vi "Pockels Cal-Calibration case logic.vi"(4 "Voltage %":u16[](array[numeric])=[0, 5, 10, 15, 20, 25, 30, 35, 40, 45, 50, 55, 60, 65, 70, 75, 80, 85, 90, 95, 100], 6 "Pockels calibration voltage steps sequence":dbl[](array[numeric])=[0.0, 0.05, 0.1, 0.15000000000000002, 0.2, 0.25, 0.3, 0.35, 0.39999999999999997, 0.44999999999999996, 0.49999999999999994, 0.5499999999999999, 0.6, 0.65, 0.7000000000000001, 0.7500000000000001, 0.8000000000000002, 0.8500000000000002, 0.9000000000000002, 0.9500000000000003, 1.0000000000000002], 7 "Number of objectives + 1":i32, 10 "Objective's name":string, 11 "Parent FOR loop's index":i32) -> (0 "error out":errorcluster, 2 "Timed out or errored out":bool, 3 "Cancel & Exit":bool, 5 "Output Strings":string[](array[string]))   [LabVIEW 2020]
panel:
  out "Cal indexes":i32[](array[numeric])
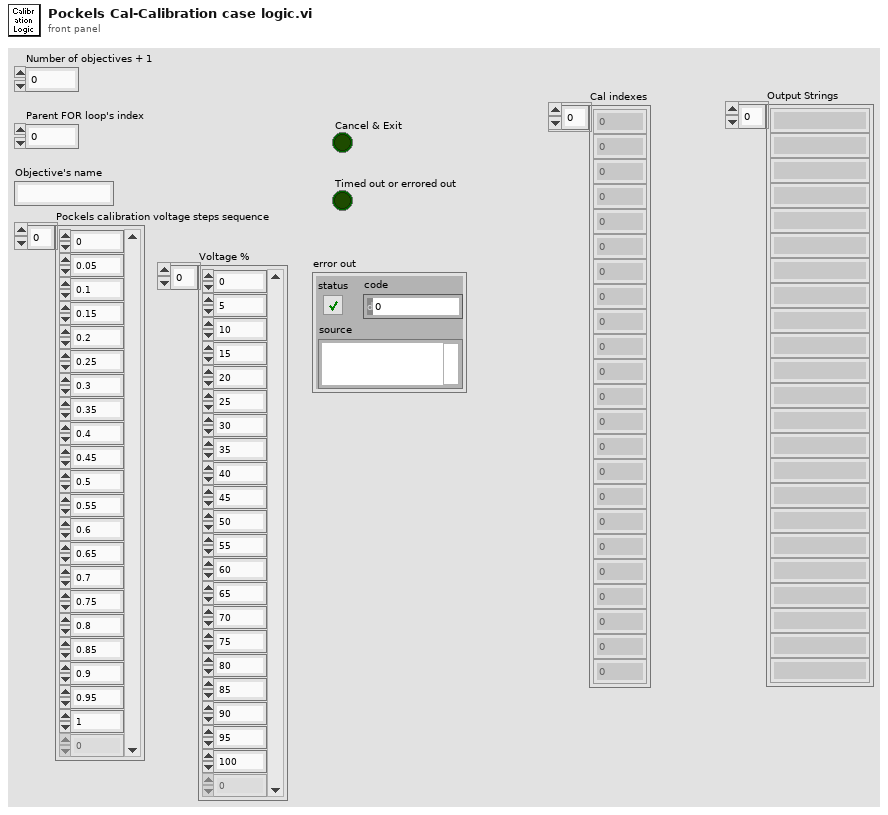
[diagram p1: front panel]
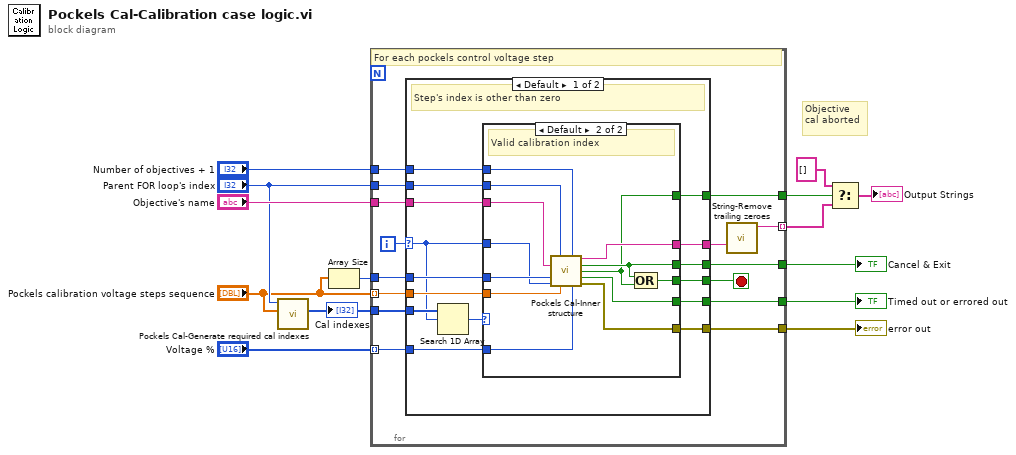
[diagram p0: block diagram]
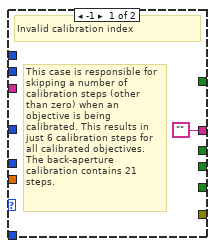
[diagram p2: hidden frame]
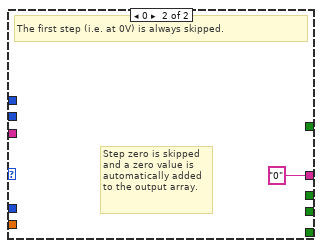
[diagram p3: hidden frame]
diagram:
  # "Objective cal aborted"
  n1 = call "Pockels Cal-Generate required cal indexes.vi"("Pockels calibration voltage steps sequence"="Pockels calibration voltage steps sequence", "Parent FOR loop's index"="Parent FOR loop's index") -> ("Required Cal indexes"=w2:i32[])  [unwired: 9 in]
  "Cal indexes" <- w2
  n2 = Array Size(array="Pockels calibration voltage steps sequence") -> (size(s)=w3:i32)
  n3 = for {
    tunnel: "Pockels calibration voltage steps sequence" -> [w23] mode=indexing
    tunnel: "Objective's name" -> [w28]
    tunnel: [w21] -> w13 mode=indexing
    tunnel: [w18] -> w6
    tunnel: w3 -> [w24]
    tunnel: [w29] -> w7
    tunnel: "Number of objectives + 1" -> [w27]
    tunnel: "Parent FOR loop's index" -> [w26]
    tunnel: [w25] -> w9
    tunnel: "Voltage %" -> [w22] mode=indexing
    tunnel: [w16] -> w11
    tunnel: w2 -> [w15]
    i -> [w19]
    stop <- w17 stop-if-true
    # "For each pockels control voltage step"
    n4 = case shown="Default" w19 {
      selector: w19 -> [w31 _]
      tunnel: [w35 _] -> w18
      tunnel: [w44 _] -> w29
      tunnel: w28 -> [w43 _]
      tunnel: w27 -> [w42 _]
      tunnel: w26 -> [w41 _]
      tunnel: [w40 _] -> w25
      tunnel: w24 -> [w39 _]
      tunnel: w23 -> [w38 _]
      tunnel: w22 -> [w37 _]
      tunnel: [w36 "0"] -> w20
      tunnel: [w34 _] -> w17
      tunnel: [w33 _] -> w16
      tunnel: w15 -> [w32 _]
      frame Default {
        # "Step's index is other than zero"
        n5 = Search 1D Array(1D array=w32, element=w31) -> (index of element=w30:i32)  [unwired: 1 in]
        n6 = case shown="Default" w30 {
          tunnel: [_ w58] -> w44
          tunnel: w43 -> [_ w57]
          tunnel: w42 -> [_ w56]
          tunnel: w41 -> [_ w55]
          tunnel: [_ w54] -> w40
          tunnel: w39 -> [_ w53]
          tunnel: w38 -> [_ w52]
          tunnel: w37 -> [_ w51]
          tunnel: ["" ("String") w50] -> w36
          tunnel: w31 -> [_ w49]
          tunnel: [_ w48] -> w35
          tunnel: [_ w47] -> w34
          tunnel: [_ w46] -> w33
          frame -1 {
            # "This case is responsible for skipping a number of calibration steps (other than zero) when an objective is being calibrated. This results in just 6 calibration steps for all calibrated objectives. The back-aperture calibration contains 21 steps."
            # "Invalid calibration index"
          }
          frame Default {
            # "Valid calibration index"
            n7 = call "Pockels Cal-Inner structure.vi"("Index of current outer loop iteraton (Index of objective +1)"=w55, "Number of outer loop iteratons"=w56, "Objective's name"=w57, "Number of voltage steps per objective"=w53, "Pockels control voltage index"=w49, "Pockels calibration voltage"=w52, "Voltage %"=w51) -> ("String"=w50:string, "Cancel & Exit"=w48:bool, "Abort this objective"=w46:bool, "Timed out or errored out"=w58:bool, "error out"=w54:errorcluster)  [unwired: 4 in]
            n8 = Compound Arithmetic op=OR(w48, w46) -> (w47:bool)
          }
        }
      }
      frame 0 {
        # "Step zero is skipped and a zero value is automatically added to the output array."
        # "The first step (i.e. at 0V) is always skipped."
      }
    }
    n9 = call <userlib>:"String-Remove trailing zeroes.vi"("String in"=w20) -> ("String out"=w21:string)  [unwired: 10 in]
  }
  "error out" <- w9
  "Timed out or errored out" <- w7
  "Cancel & Exit" <- w6
  n10 = Select(t=string[] [], s=w11, f=w13) -> (s? t:f=→"Output Strings":string[])
